vi "CombineSignals.vi"(8 "Old signal":waveform(dbl)[](array[waveform]), 11 "New signal":waveform(dbl)[](array[waveform])) -> (1 "Ch 2":waveform(dbl)(graph), 3 "Ch 1":waveform(dbl)(graph))   [LabVIEW 2022 SP3]
uses:
  <vilib>/Waveform/WDTOps.llb/WDT Append Waveforms DBL.vi
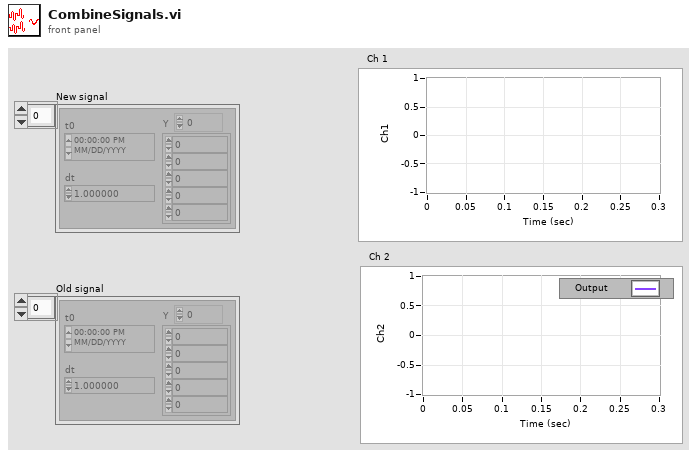
[diagram p1: front panel]
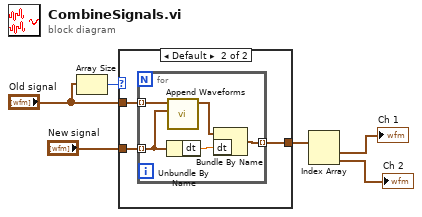
[diagram p0: block diagram]
diagram:
  n1 = Array Size(array="Old signal") -> (size(s)=w6:i32)
  n2 = case shown="Default" w6 {
    tunnel: "New signal" -> [w7 w10]
    tunnel: "Old signal" -> [_ w9]
    tunnel: [w7 w8] -> w3
    frame 0 {
    }
    frame Default {
      n3 = for {
        tunnel: w10 -> [w12] mode=indexing
        tunnel: [w13] -> w8 mode=indexing
        tunnel: w9 -> [w15] mode=indexing
        n4 = Unbundle By Name(w12) -> ("dt"=w11:dbl)
        n5 = call-poly <vilib>:"Append Waveforms.vi"("waveform B"=w12, "waveform A"=w15) -> ("waveform out"=w14:waveform(dbl))  [unwired: 8 in, 1 out]
        n6 = Bundle By Name(cluster=w14, "dt"=w11) -> (w13:waveform(dbl))
      }
    }
  }
  n7 = Index Array(array=w3) -> (element #1=→"Ch 1":waveform(dbl), element #2=→"Ch 2":waveform(dbl))  [unwired: 2 in]
